vi "First_Code_EV3.vi"() -> ()   [LabVIEW 2012]
uses:
  <vilib>/NXT/Subs/MotorOutput.ctl
  SubVIs/LVPresent_Globals.vi
panel:
  in  "Run":bool
  in  "Abort":bool
  in  "?":bool
  # "Writing LabVIEW Code\n\nMake sure that the EV3 is connected to your computer via a USB cord. Click the Run button - does the car move?  In order to stop the program, click the Abort button.  Click the Open button to open this program in LabVIEW."
  # "Abort"
  # "Run"
  # "Click the open button to open the program and see more helpful tips!"
  # "Once you open the program, test out the following, and see if you can move and break things:\n          -Change the number 75 to any value between -100 and 100, and run it again.  \n            What happens when this value is negative? \n          -Try changing the Port - from All Ports to Port A or B (depending on what \n            ports you have connected to the motors)."
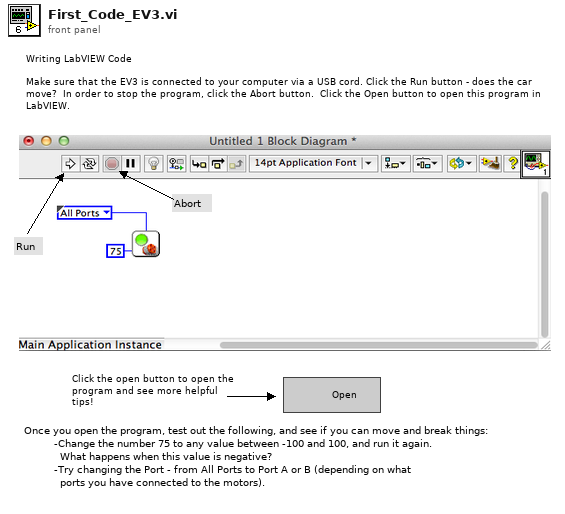
[diagram p1: front panel]
types:
  T1 = typedef "MotorOutput.ctl" = u8
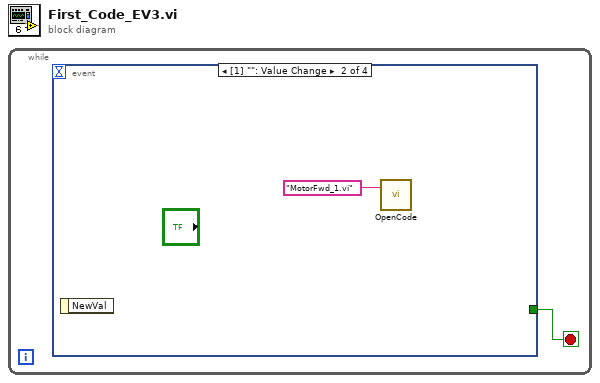
[diagram p0: block diagram]
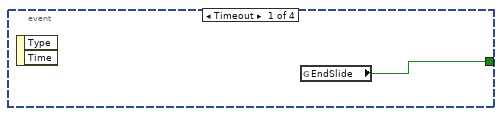
[diagram p2: hidden frame]
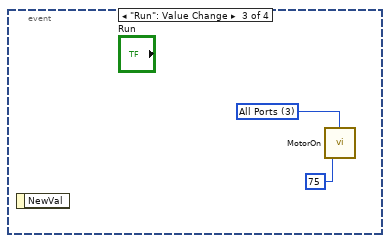
[diagram p3: hidden frame]
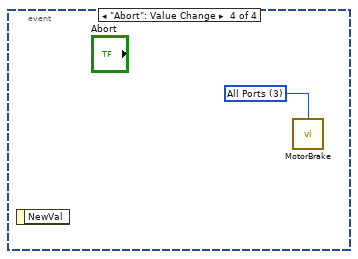
[diagram p4: hidden frame]
diagram:
  n1 = while {
    stop <- w1 stop-if-true
    n2 = event shown="[1] \"\": Value Change" {
      selector: _ -> [_ _ _ _]
      dyn-events: _ -> [_ _ _ _]
      timeout: _ -> [_ _ _ _]
      tunnel: [w2 _ _ _] -> w1
      event Timeout {
        n3 = event-data() -> ()  [unwired: 1 in, 2 out]
        n4 = global read "LVPresent_Globals.vi" "EndSlide"() -> (w2:bool)
      }
      event Value Change {
        n5 = event-data() -> ()  [unwired: 1 in, 1 out]
        n6 = call "OpenCode.vi"("Code name"="MotorFwd_1.vi") -> ()  [unwired: 3 in]
      }
      event "Run": Value Change {
        w4 = T1 3 items=["Port A"=0, "Port B"=1, "Port C"=2, "Ports A & B"=4, "Ports A & C"=5, "Ports B & C"=6, "All Ports"=3] ("Output Port (All Ports)")
        n7 = event-data() -> ()  [unwired: 1 in, 1 out]
        n8 = call <vilib>:"MotorOn.vi"("Power (75)"=75, "Output Port (All Ports)"=w4) -> ()  [unwired: 2 in, 1 out]
      }
      event "Abort": Value Change {
        w6 = T1 3 items=["Port A"=0, "Port B"=1, "Port C"=2, "Ports A & B"=4, "Ports A & C"=5, "Ports B & C"=6, "All Ports"=3] ("Port (All Ports)")
        n9 = event-data() -> ()  [unwired: 1 in, 1 out]
        n10 = call <vilib>:"MotorBrake.vi"("Port (All Ports)"=w6) -> ()  [unwired: 3 in, 1 out]
      }
    }
  }
